vi "SpinCoaterArray2String_v02.vi"(3 "Time Start":dbl[unit], 4 "Program Spin Coater\nSpeed (rpm)          Time (s)":dbl[][](array[numeric])) -> (1 "remote control String":string)   [LabVIEW 2018]
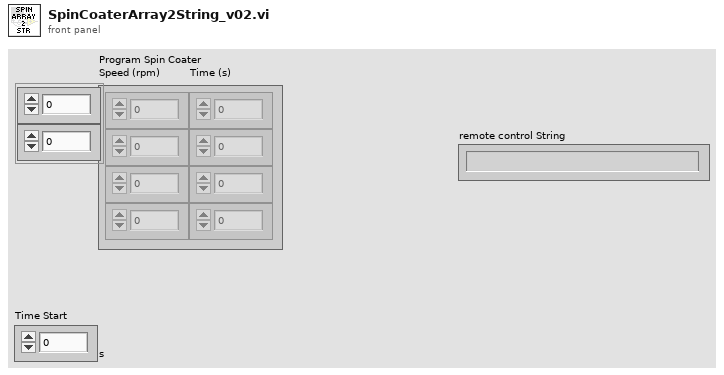
[diagram p1: front panel]
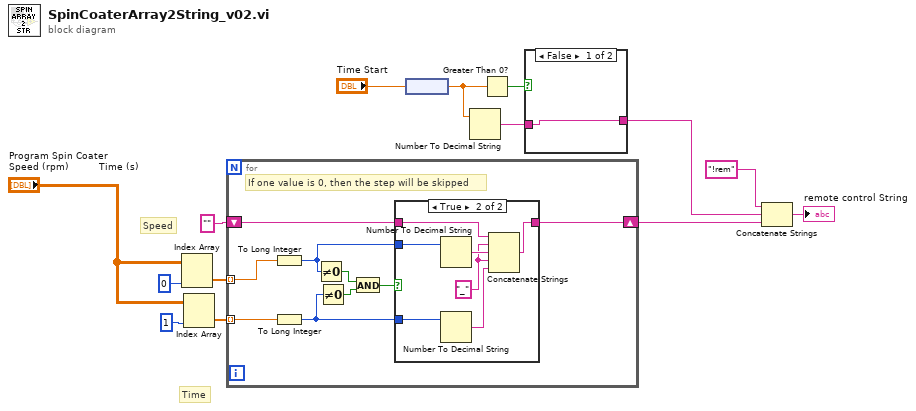
[diagram p0: block diagram]
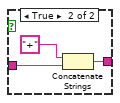
[diagram p2: hidden frame]
diagram:
  # "Time"
  # "Speed"
  n1 = Index Array(array="Program Spin Coater\nSpeed (rpm)          Time (s)", index (col)=0 ("disabled index (col)")) -> (element=w11:dbl[])  [unwired: 1 in]
  n2 = Index Array(array="Program Spin Coater\nSpeed (rpm)          Time (s)", index (col)=1 ("disabled index (col)")) -> (element=w10:dbl[])  [unwired: 1 in]
  n3 = for {
    tunnel: w11 -> [w20] mode=indexing
    tunnel: w10 -> [w19] mode=indexing
    shift-right: [w15] -> w1
    shift-left: "" ("string") -> [w16]
    # "If one value is 0, then the step will be skipped"
    n4 = To Long Integer(number=w20) -> (32bit integer=w18:i32)
    n5 = To Long Integer(number=w19) -> (32bit integer=w17:i32)
    n6 = Not Equal To 0?(x=w18) -> (x != 0?=w23:bool)
    n7 = Not Equal To 0?(x=w17) -> (x != 0?=w22:bool)
    n8 = And(x=w23, y=w22) -> (x .and. y?=w21:bool)
    n9 = case shown="True" w21 {
      tunnel: w18 -> [_ w31]
      tunnel: w17 -> [_ w30]
      tunnel: w16 -> [w24 w26]
      tunnel: [w24 w25] -> w15
      frame False {
      }
      frame True {
        w27 = "_" ("string")
        n10 = Number To Decimal String(number=w31) -> (decimal integer string=w29:string)  [unwired: 1 in]
        n11 = Number To Decimal String(number=w30) -> (decimal integer string=w28:string)  [unwired: 1 in]
        n12 = Concatenate Strings(w26, w27, w29, w27, w28) -> (w25:string)
      }
    }
  }
  n13 = node("Time Start") -> (w5:dbl)
  n14 = Number To Decimal String(number=w5) -> (decimal integer string=w4:string)  [unwired: 1 in]
  n15 = Greater Than 0?(x=w5) -> (x > 0?=w6:bool)
  n16 = case shown="False" w6 {
    tunnel: w4 -> [w32 w34]
    tunnel: [w32 w33] -> w3
    frame False {
    }
    frame True {
      n17 = Concatenate Strings("+", w34) -> (w33:string)
    }
  }
  n18 = Concatenate Strings("!rem" ("string"), w3, w1) -> (→"remote control String":string)
